vi "02datos_multiequipo.vi"(3 "Nº equipo":i32, 4 "EE 492":T3(array[cluster]), 5 "Config Equipos":T2(array[cluster]) {"Ref PD" max=10000 step=1; "Med Princ" items=["1", "2", "3", "4", "5", "6", "7", "8", "9", "10", "11", "12", "13", "14", "15", "16", "17", "18", "19", "20", "21", "22", "23", "24", "25", "26", "27", "28", "29", "30", "31", "32"]}) -> (1 "Medicion Eq":T1)   [LabVIEW 2010]
panel:
  out "error out":errorcluster
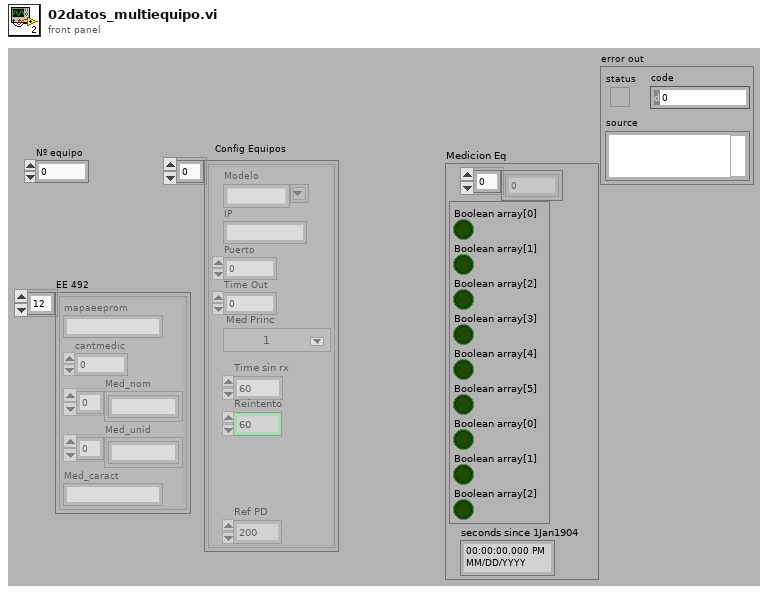
[diagram p1: front panel]
types:
  T1 = cluster{dbl[], cluster{"Boolean array[0]":bool, "Boolean array[1]":bool, "Boolean array[2]":bool, "Boolean array[3]":bool, "Boolean array[4]":bool, "Boolean array[5]":bool, "Boolean array[0]":bool, "Boolean array[1]":bool, "Boolean array[2]":bool}, "seconds since 1Jan1904":timestamp}
  T2 = cluster{"Modelo":string, "IP":string, "Puerto":u16, "Time Out":u16, "Med Princ":u16, "Time sin rx":u16, "Reintento":u16, "Ref PD":u16}[]
  T3 = cluster{"mapaeeprom":string, "cantmedic":u8, "Med_nom":string[], "Med_unid":string[], "Med_caract":string}[]
  T4 = cluster{"mapaeeprom":string, "cantmedic":u8, "Med_nom":string[], "Med_unid":string[], "Med_caract":string}
  T5 = cluster{"Boolean array[0]":bool, "Boolean array[1]":bool, "Boolean array[2]":bool, "Boolean array[3]":bool, "Boolean array[4]":bool, "Boolean array[5]":bool, "Boolean array[0]":bool, "Boolean array[1]":bool, "Boolean array[2]":bool}
  T6 = cluster{"Modelo":string, "IP":string, "Puerto":u16, "Time Out":u16, "Med Princ":u16, "Time sin rx":u16, "Reintento":u16, "Ref PD":u16}
  T7 = cluster{"unsigned byte array[0]":u8, "unsigned byte array[1]":u8}
  T8 = cluster{"Boolean array[0]":bool, "Boolean array[1]":bool, "Boolean array[2]":bool}
  T9 = cluster{"Boolean array[0]":bool, "Boolean array[1]":bool, "Boolean array[2]":bool, "Boolean array[3]":bool, "Boolean array[4]":bool, "Boolean array[5]":bool}
  T10 = cluster{"Boolean array[0]":bool, "Boolean array[0]":bool, "Boolean array[0]":bool, "Boolean array[0]":bool, "Boolean array[0]":bool, "Boolean array[0]":bool, "Boolean array[0]":bool, "Boolean array[0]":bool, "Boolean array[0]":bool}
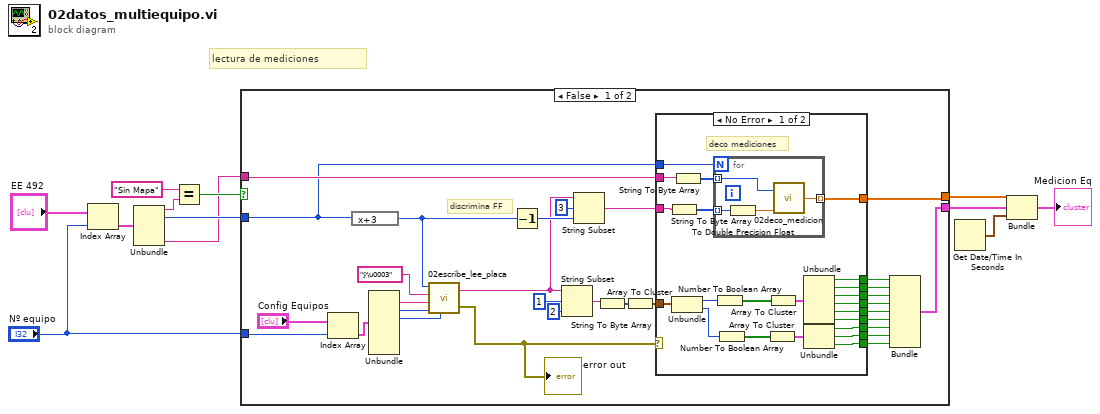
[diagram p0: block diagram]
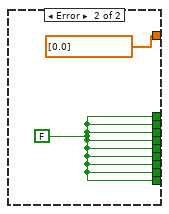
[diagram p2: hidden frame]
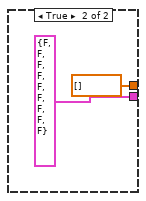
[diagram p3: hidden frame]
diagram:
  # "lectura de mediciones"
  n1 = Index Array(array="EE 492", index="Nº equipo") -> (element=w12:T4)
  n2 = Unbundle(w12) -> ("mapaeeprom"=w10:string, "cantmedic"=w11:u8, "Med_caract"=w7:string)  [unwired: 2 out]
  n3 = Equal?(x="Sin Mapa", y=w10) -> (x = y?=w8:bool)
  n4 = case shown="False" w8 {
    tunnel: [w24 sgl[] []] -> w5
    tunnel: w11 -> [w21 _]
    tunnel: w7 -> [w22 _]
    tunnel: [w27 T5 {"Boolean array[0]"=FALSE, "Boolean array[1]"=FALSE, "Boolean array[2]"=FALSE, "Boolean array[3]"=FALSE, "Boolean array[4]"=FALSE, "Boolean array[5]"=FALSE, "Boolean array[0]"=FALSE, "Boolean array[1]"=FALSE, "Boolean array[2]"=FALSE}] -> w4
    tunnel: "Nº equipo" -> [w17 _]
    frame False {
      # "discrimina FF"
      n5 = Index Array(array="Config Equipos", index=w17) -> (element=w19:T6)
      n6 = expression code="x+3"(w21) -> (w25:u8)
      n7 = Unbundle(w19) -> ("IP"=w15:string, "Puerto"=w14:u16, "Time Out"=w13:u16)  [unwired: 5 out]
      n8 = call "02escribe_lee_placa.vi"("cantmedic"=w25, "comando"="ÿ\u0003" ("string to write"), "IP"=w15, "Puerto"=w14, "Time Out"=w13) -> ("DATA"=w39:string, "error out"=w16:errorcluster)
      "error out" <- w16
      n9 = Decrement(x=w25) -> (x-1=w43:u8)
      n10 = String Subset(string=w39, offset (0)=1, length (rest)=2 ("length (rest)")) -> (substring=w26:string)
      n11 = String Subset(string=w39, offset (0)=3, length (rest)=w43) -> (substring=w23:string)
      n12 = String To Byte Array(string=w26) -> (unsigned byte array=w28:u8[])
      n13 = Array To Cluster(array=w28) -> (cluster=w29:T7)
      n14 = case shown="No Error" w16 {
        tunnel: [w65 w70] -> w38
        tunnel: [w64 w70] -> w37
        tunnel: [w63 w70] -> w36
        tunnel: [w62 w70] -> w35
        tunnel: [w61 w70] -> w34
        tunnel: [w60 w70] -> w33
        tunnel: [w59 w70] -> w32
        tunnel: [w58 w70] -> w31
        tunnel: [w57 w70] -> w30
        tunnel: w29 -> [w56 _]
        tunnel: [w49 dbl[] [0.0]] -> w24
        tunnel: w23 -> [w47 _]
        tunnel: w22 -> [w45 _]
        tunnel: w21 -> [w48 _]
        frame No Error {
          # "deco mediciones"
          n15 = String To Byte Array(string=w47) -> (unsigned byte array=w46:u8[])
          n16 = Unbundle(w56) -> ("unsigned byte array[0]"=w52:u8, "unsigned byte array[1]"=w51:u8)
          n17 = String To Byte Array(string=w45) -> (unsigned byte array=w44:u8[])
          n18 = for {
            N: w48 -> [_]
            tunnel: [w69] -> w49 mode=indexing
            tunnel: w46 -> [w67] mode=indexing
            tunnel: w44 -> [w66] mode=indexing
            n19 = To Double Precision Float(number=w67) -> (double precision float=w68:dbl)
            n20 = call "02deco_medicion.vi"("medicion"=w68, "caract"=w66) -> ("Numeric"=w69:dbl)
          }
          n21 = Number To Boolean Array(number=w52) -> (Boolean array=w53:bool[])
          n22 = Number To Boolean Array(number=w51) -> (Boolean array=w50:bool[])
          n23 = Array To Cluster(array=w50) -> (cluster=w54:T8)
          n24 = Array To Cluster(array=w53) -> (cluster=w55:T9)
          n25 = Unbundle(w55) -> ("Boolean array[0]"=w57:bool, "Boolean array[1]"=w58:bool, "Boolean array[2]"=w59:bool, "Boolean array[3]"=w60:bool, "Boolean array[4]"=w61:bool, "Boolean array[5]"=w62:bool)
          n26 = Unbundle(w54) -> ("Boolean array[0]"=w63:bool, "Boolean array[1]"=w64:bool, "Boolean array[2]"=w65:bool)
        }
        frame Error {
          w70 = FALSE ("Boolean array[0]")
        }
      }
      n27 = Bundle("Boolean array[0]"=w30, "Boolean array[0]"=w31, "Boolean array[0]"=w32, "Boolean array[0]"=w33, "Boolean array[0]"=w34, "Boolean array[0]"=w35, "Boolean array[0]"=w36, "Boolean array[0]"=w37, "Boolean array[0]"=w38) -> (w27:T10)  [unwired: 1 out]
    }
    frame True {
    }
  }
  n28 = Get Date/Time In Seconds() -> (seconds since 1Jan1904=w6:timestamp)
  n29 = Bundle(w5, w4, "seconds since 1Jan1904"=w6) -> (→"Medicion Eq":T1)  [unwired: 1 out]
